vi "GA_Single Breed.vi"(6 "Parameters":T2={"Population size"=100, "Generations no."=500, "Significant digits"=4, "Crossover probabality"=0.85, "Mutation mode"=enum."one-point, fixed rate", "Use Gray code?"=FALSE, "Mutation rate"=0.05, "Min mutation rate"=0.0005, "Max mutation rate"=0.25, "Reproduction plan"=enum."Steady-state-replace-worst", "Elitism"=FALSE, "Fmax"=1} {"Max mutation rate" min=0.0 max=1.0; "Min mutation rate" min=0.0 max=1.0; "Mutation rate" min=0.0 max=1.0; "Crossover probabality" min=0.0 max=1.0; "Significant digits" min=1; "Generations no." min=1; "Population size" min=1}, 11 "Population in":T1) -> (0 "Offsprings":i32[][](array[numeric]), 3 "Population out":T1)   [LabVIEW 2016, in "Optimal Frequency Bands Search.lvlib" / "GeneticAlgorithm.lvlib"]
doc: "Процедура скрещивания (кроссовера). Выбор двух предков из популяции и порождение двух потомков"
uses:
  GeneticAlgorithm.lvlib
  GA_tParameters.ctl
  GA_tPopulation.ctl
panel:
  # "This VI is a part of BCI Design library, http://www.ru-bci.org \nCopyright © 2020, Sotnikov Peter, All rights reserved. License: CC BY-NC 4.0"
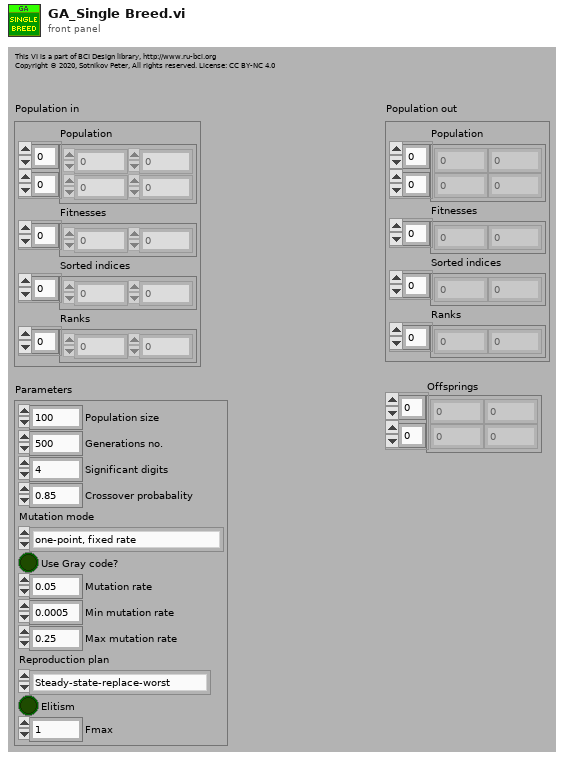
[diagram p1: front panel]
types:
  T1 = typedef "Optimal Frequency Bands Search.lvlib/GeneticAlgorithm.lvlib/GA_tPopulation.ctl" = cluster{"Population":i32[][], "Fitnesses":dbl[], "Sorted indices":i32[], "Ranks":i32[]}
  T2 = typedef "Optimal Frequency Bands Search.lvlib/GeneticAlgorithm.lvlib/GA_tParameters.ctl" = cluster{"Population size":i32, "Generations no.":i32, "Significant digits":i32, "Crossover probabality":dbl, "Mutation mode":enum16{"one-point, fixed rate", "one-point, fitness-adjustable rate", "one-point, distance-adjustable rate"}, "Use Gray code?":bool, "Mutation rate":dbl, "Min mutation rate":dbl, "Max mutation rate":dbl, "Reproduction plan":enum16{"Full generational replacement", "Steady-state-replace-random", "Steady-state-replace-worst"}, "Elitism":bool, "Fmax":i32}
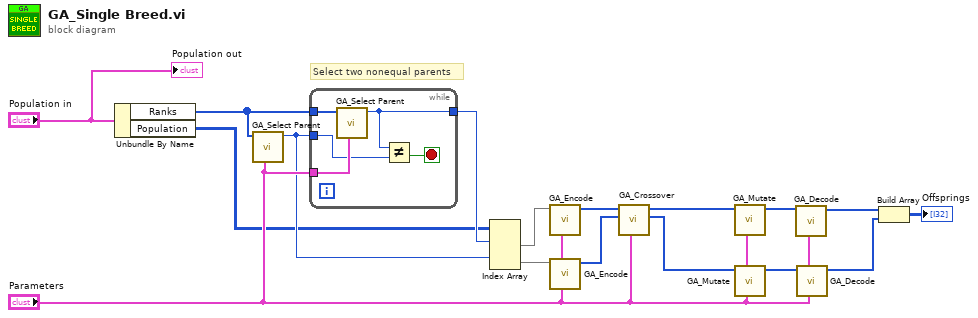
[diagram p0: block diagram]
diagram:
  # "Select two nonequal parents"
  n1 = Unbundle By Name("Population in") -> ("Ranks"=w5:i32[], "Population"=w4:i32[][])
  n2 = call "GA_Select Parent.vi"("Parameters"="Parameters", "Ranks"=w5) -> ("Parent index"=w8:i32)  [unwired: 9 in]
  n3 = while {
    tunnel: w8 -> [w20]
    tunnel: w5 -> [w22]
    tunnel: "Parameters" -> [w21]
    tunnel: [w18] -> w7
    stop <- w19 stop-if-true
    n4 = call "GA_Select Parent.vi"("Parameters"=w21, "Ranks"=w22) -> ("Parent index"=w18:i32)  [unwired: 9 in]
    n5 = Not Equal?(x=w18, y=w20) -> (x != y?=w19:bool)
  }
  n6 = Index Array(array=w4, index (row) #1=w7, index (row) #2=w8) -> (element #1=w10:i32[], element #2=w9:i32[])  [unwired: 2 in]
  n7 = call "GA_Encode.vi"("Parameters"="Parameters", "Phenotype"=w10) -> ("Genotype"=w12:i8[])  [unwired: 9 in]
  n8 = call "GA_Encode.vi"("Parameters"="Parameters", "Phenotype"=w9) -> ("Genotype"=w11:i8[])  [unwired: 9 in]
  n9 = call "GA_Crossover.vi"("Parameters"="Parameters", "Genotype 2"=w11, "Genotype 1"=w12) -> ("Offspring 2"=w13:i8[], "Offspring 1"=w14:i8[])  [unwired: 7 in]
  n10 = call "GA_Mutate.vi"("Parameters"="Parameters", "Genotype in"=w14) -> ("Genotype out"=w15:i8[])  [unwired: 9 in]
  n11 = call "GA_Mutate.vi"("Parameters"="Parameters", "Genotype in"=w13) -> ("Genotype out"=w16:i8[])  [unwired: 9 in]
  n12 = call "GA_Decode.vi"("Parameters"="Parameters", "Genotype"=w15) -> ("Phenotype"=w2:i32[])  [unwired: 9 in]
  n13 = call "GA_Decode.vi"("Parameters"="Parameters", "Genotype"=w16) -> ("Phenotype"=w1:i32[])  [unwired: 9 in]
  n14 = Build Array(w2, w1) -> (→"Offsprings":i32[][])
  "Population out" <- "Population in"
